vi "PJ1_สไลด์.vi"() -> ()   [LabVIEW 2024]
uses:
  <vilib>/express/express analysis/Spectral/XNode/ExpressSpectralMeasurementsBlockNode.xnode
  <vilib>/express/express analysis/Spectral/Block/exnSpectralBlock spectral measurements PSD poly.vi
  <vilib>/express/express analysis/Spectral/Block/exnSpectralBlock spectral measurements PSD DDT.vi
  <vilib>/Instr/_visa.llb/VISA Configure Serial Port (Instr).vi
panel:
  out "Numeric":i32
  in  "Upper Cut-Off":dbl=40.0
  out "PSD":dynamicdata(graph)
  out "PSD MAX":dbl
  out "Index ที่มากที่สุด":i32
  out "max value":dbl
  out "B 18+1":dbl
  out "N 18+1":dbl
  in  "Aj 18+1":dbl
  out "B 18+1":dbl
  out "PSD 18+1":dbl
  out "B 18":dbl
  out "N 18":dbl
  in  "Aj 18":dbl
  out "B 18":dbl
  out "PSD 18":dbl
  out "B 18-1":dbl
  out "N 18-1":dbl
  in  "Aj 18-1":dbl
  out "B 18-1":dbl
  out "PSD 18-1":dbl
  out "9 Hz":dbl[](array[numeric])
  out "Max Index 9":i32
  out "PSD max 9":dbl
  out "PSD 9-1":dbl
  out "B 9-1":dbl
  in  "Aj 9-1":dbl
  out "N 9-1":dbl
  out "B 9-1":dbl
  out "PSD 9":dbl
  out "B 9":dbl
  in  "Aj 9":dbl
  out "N 9":dbl
  out "B 9":dbl
  out "PSD 9+1":dbl
  out "B 9+1":dbl
  in  "Aj 9+1":dbl
  out "N 9+1":dbl
  out "B 9+1":dbl
  out "8 Hz":dbl[](array[numeric])
  out "Max Index 8":i32
  out "PSD max 8":dbl
  out "B 16+1":dbl
  out "N 16+1":dbl
  in  "Aj  16+1":dbl
  out "B 16+1":dbl
  out "PSD  16+1":dbl
  out "B 16":dbl
  out "N  16":dbl
  in  "Aj  16":dbl
  out "B 16":dbl
  out "PSD  16":dbl
  out "B 16-1":dbl
  out "N  16-1":dbl
  in  "Aj   16-1":dbl
  out "B   16-1":dbl
  out "PSD 16-1":dbl
  out "B 8+1":dbl
  out "N 8+1":dbl
  in  "Aj  8+1":dbl
  out "B  8+1":dbl
  out "PSD 8+1":dbl
  out "B 8":dbl
  out "N  8":dbl
  in  "Aj  8":dbl
  out "B  8":dbl
  out "PSD 8":dbl
  out "B 8-1":dbl
  out "N  8-1":dbl
  in  "Aj  8-1":dbl
  out "B  8-1":dbl
  out "PSD 8-1":dbl
  out "PSD 14+1":dbl
  out "B 14+1":dbl
  in  "Aj 14+1":dbl
  out "N 14+1":dbl
  out "B 14+1":dbl
  out "PSD 14":dbl
  out "B 14":dbl
  in  "Aj 14":dbl
  out "N 14":dbl
  out "B 14":dbl
  out "PSD 14-1":dbl
  out "B 14-1":dbl
  in  "Aj 14-1":dbl
  out "N 14-1":dbl
  out "B 14-1":dbl
  out "PSD7+1":dbl
  out "B7+1":dbl
  in  "Aj7+1":dbl
  out "N7+1":dbl
  out "B7+1":dbl
  out "PSD 7":dbl
  out "B 7":dbl
  in  "Aj 7":dbl
  out "N7":dbl
  out "B7":dbl
  out "7 Hz":dbl[](array[numeric])
  out "Max Index 7":i32
  out "PSD max 7":dbl
  out "PSD 7-1":dbl
  out "B 7-1":dbl
  in  "Aj 7-1":dbl
  out "N7-1":dbl
  out "B7-1":dbl
  out "B12-1":dbl
  out "N12-1":dbl
  in  "Aj 12-1":dbl
  out "B 12-1":dbl
  out "PSD 12-1":dbl
  out "B12":dbl
  out "N12":dbl
  in  "Aj 12":dbl
  out "B12":dbl
  out "PSD 12":dbl
  out "B12+1":dbl
  out "N12+1":dbl
  in  "Aj 12+1":dbl
  out "B 12+1":dbl
  out "PSD 12+1":dbl
  out "B6+1":dbl
  out "N6+1":dbl
  in  "Aj 6+1":dbl
  out "B 6+1":dbl
  out "PSD 6+1":dbl
  out "B6":dbl
  out "N6":dbl
  in  "Aj 6":dbl
  out "B6":dbl
  out "PSD 6":dbl
  out "PSD 6-1":dbl
  out "6 Hz":dbl[](array[numeric])
  out "Max Index 6":i32
  out "PSD max 6":dbl
  out "B 6-1":dbl
  in  "Aj 6-1":dbl
  out "N6-1":dbl
  out "B6-1":dbl
  in  "Baseline":bool
  out "appended array":dbl[][](array[numeric])
  out "Filtered Signal":dynamicdata(graph)
  in  "Lower Cut-Off":dbl=1.0
  out "data":dynamicdata(graph) caption="Raw Data"
  in  "number of samples":i32=1000
  in  "rate":dbl=200.0 min=200.0 max=200.0
  out "?":bool
  out "?":bool
  out "?":bool
  out "?":bool
  out "?":bool
  out "?":bool
  out "?":bool
  out "?":bool
  out "?":bool
  out "?":bool
  out "?":bool=TRUE
  out "?":bool=TRUE
  out "?":bool=TRUE
  out "?":bool=TRUE
  out "?":bool=TRUE
  out "?":bool=TRUE
  out "?":bool=TRUE
  out "?":bool=TRUE
  out "?":bool=TRUE
  out "?":bool=TRUE
  out "?":bool
  out "?":bool
  out "?":bool
  out "?":bool
  out "?":bool
  out "?":bool
  out "?":bool
  out "?":bool
  out "?":bool
  out "?":bool
  out "?":bool=TRUE
  out "?":bool=TRUE
  out "?":bool=TRUE
  out "?":bool=TRUE
  out "?":bool=TRUE
  out "?":bool=TRUE
  out "?":bool=TRUE
  out "?":bool=TRUE
  out "?":bool=TRUE
  out "?":bool=TRUE
  out "?":bool
  out "?":bool
  out "?":bool
  out "?":bool
  out "?":bool
  out "?":bool
  out "?":bool
  out "?":bool
  out "?":bool
  out "?":bool
  out "?":bool=TRUE
  out "?":bool=TRUE
  out "?":bool=TRUE
  out "?":bool=TRUE
  out "?":bool=TRUE
  out "?":bool=TRUE
  out "?":bool=TRUE
  out "?":bool=TRUE
  out "?":bool=TRUE
  out "?":bool=TRUE
  out "?":bool
  out "?":bool
  out "?":bool
  out "?":bool
  out "?":bool
  out "?":bool
  out "?":bool
  out "?":bool
  out "?":bool
  out "?":bool
  out "?":bool=TRUE
  out "?":bool=TRUE
  out "?":bool=TRUE
  out "?":bool=TRUE
  out "?":bool=TRUE
  out "?":bool=TRUE
  out "?":bool=TRUE
  out "?":bool=TRUE
  out "?":bool=TRUE
  out "?":bool=TRUE
  out "9 HZ":bool
  out "8 HZ":bool
  out "6 HZ":bool
  out "7 HZ":bool
  in  "Tab Control":enum32{"MENU", "COMMU", "CALL", "ELEC"}(tab)
  out "555":bool
  in  "ELEC":bool
  in  "MENU 3":bool
  in  "CALL":bool
  in  "COMMU":bool
  in  "start":bool
  in  "Text3":bool
  in  "Text2":bool
  out "String":string
  in  "Text1":bool
  in  "send":bool
  in  "Back 2":bool
  in  "Back 3":bool
  in  "1 3":bool
  in  "1 2":bool
  in  "1":bool
  out "String 2":string
  in  "SOS CALLING":bool
  in  "Blank Button 14":bool
  in  "LED":bool
  in  "Blank Button 12":bool
  in  "Back 4":bool
  in  "VISA resource name":refnum<visa-resource-name>
  # "Tel."
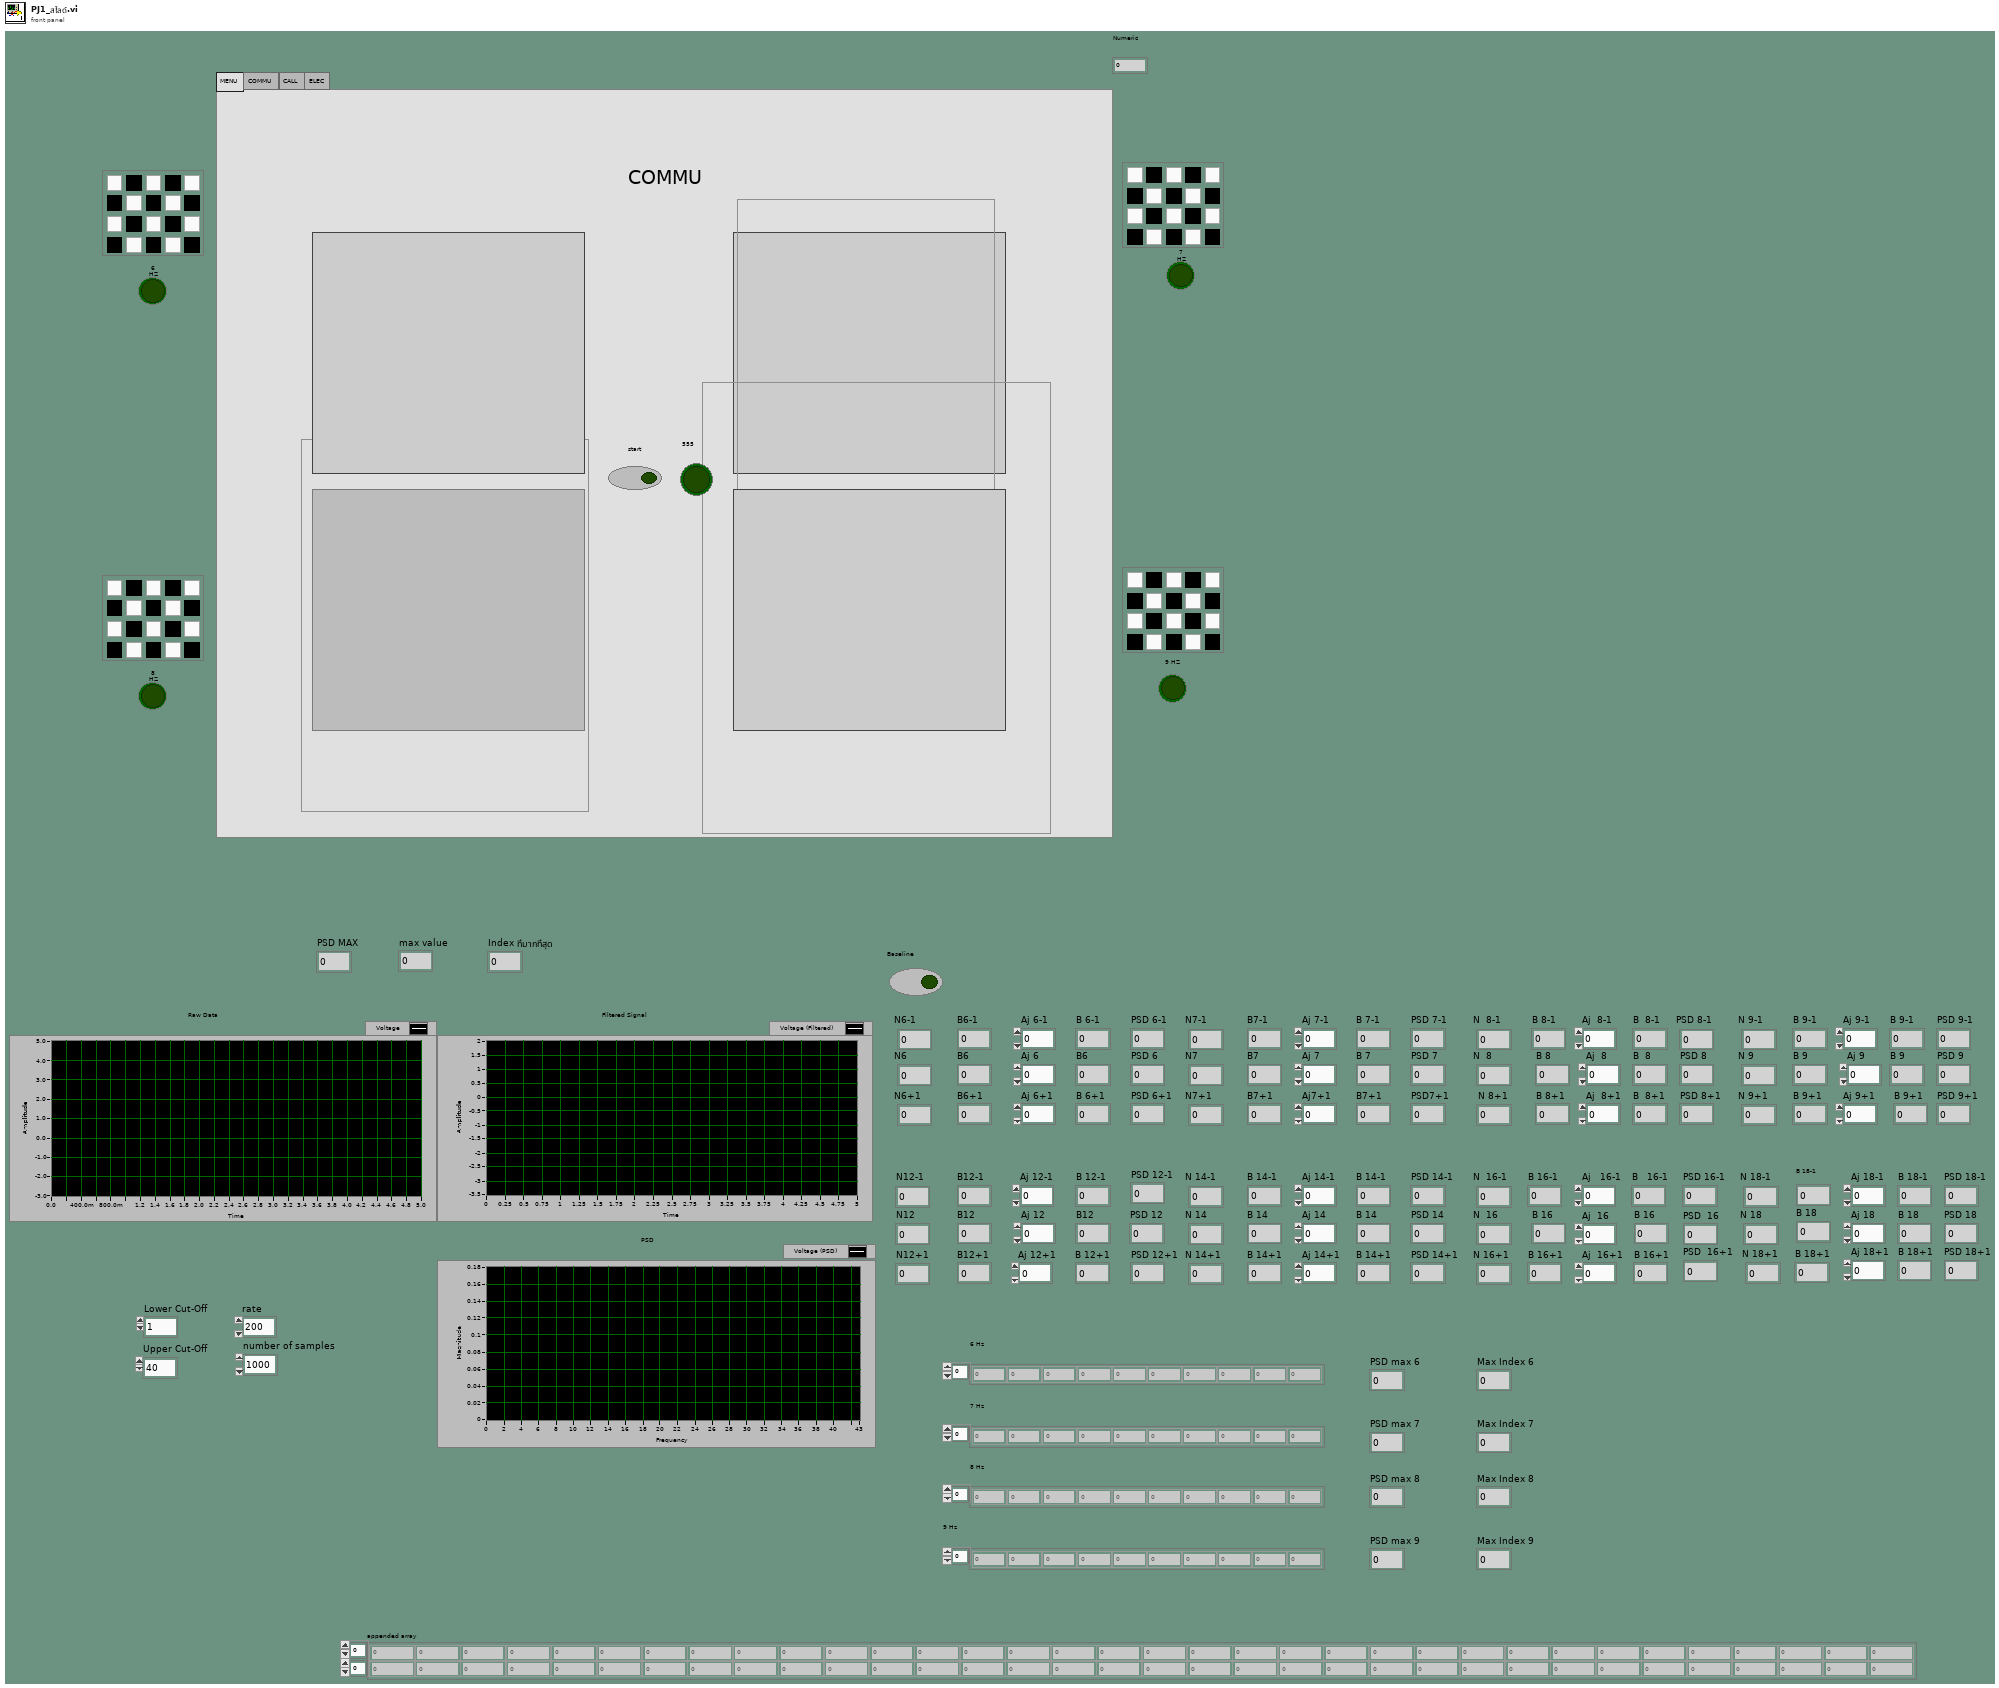
[diagram p1: front panel]
types:
  T1 = cluster{"averaging mode":u16, "weighting mode":u16, "number of averages":u32}
  T2 = cluster{"dB On (F)":bool, "unwrap phase (F)":bool, "convert to degree (F)":bool}
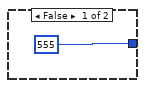
[diagram p3: hidden frame]
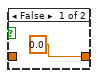
[diagram p4: hidden frame]
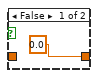
[diagram p6: hidden frame]
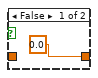
[diagram p8: hidden frame]
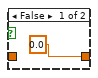
[diagram p10: hidden frame]
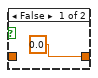
[diagram p12: hidden frame]
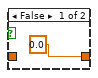
[diagram p14: hidden frame]
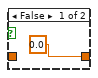
[diagram p16: hidden frame]
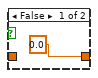
[diagram p18: hidden frame]
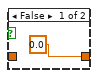
[diagram p20: hidden frame]
diagram:
  (unwired) FALSE
  n1 = while {
    stop <- FALSE stop-if-true
    n2 = event shown="[1] \"COMMU\": Value Change" {
      selector: _ -> [_ _ _ _ _ _ _]
      dyn-events: _ -> [_ _ _ _ _ _ _]
      timeout: _ -> [_ _ _ _ _ _ _]
      event Timeout {
        n3 = event-data() -> ()  [unwired: 1 in, 3 out]
      }
      event "COMMU": Value Change {
        n4 = event-data() -> ()  [unwired: 1 in, 6 out]
        n5 = local write "Tab Control"(enum32{"TAB 1", "TAB 2", "TAB 3", "TAB 4"}."TAB 2" ("Tab Control")) -> ()
      }
      event #2 (no event record) {
        n6 = event-data() -> ()  [unwired: 1 in, 6 out]
        n7 = local write "Tab Control"(enum32{"TAB 1", "TAB 2", "TAB 3", "TAB 4"}."TAB 1" ("Tab Control")) -> ()
      }
      event "CALL": Value Change {
        n8 = event-data() -> ()  [unwired: 1 in, 6 out]
        n9 = local write "Tab Control"(enum32{"TAB 1", "TAB 2", "TAB 3", "TAB 4"}."TAB 3" ("Tab Control")) -> ()
      }
      event "MENU 3": Value Change {
        n10 = event-data() -> ()  [unwired: 1 in, 6 out]
        n11 = local write "Tab Control"(enum32{"TAB 1", "TAB 2", "TAB 3", "TAB 4"}."TAB 4" ("Tab Control")) -> ()
      }
      event "ELEC": Value Change {
        n12 = event-data() -> ()  [unwired: 1 in, 6 out]
        n13 = local write "Tab Control"(enum32{"TAB 1", "TAB 2", "TAB 3", "TAB 4"}."TAB 4" ("Tab Control")) -> ()
      }
      event "Back 4": Value Change {
        n14 = event-data() -> ()  [unwired: 1 in, 6 out]
        n15 = local write "Tab Control"(enum32{"TAB 1", "TAB 2", "TAB 3", "TAB 4"}."TAB 1" ("Tab Control")) -> ()
      }
    }
  }
  n16 = while {
    shift-right: [w16] -> _
    shift-left: "" -> [w18]
    stop <- FALSE stop-if-true
    n17 = event shown="[3] \"Back 3\": Value Change" {
      selector: _ -> [_ _ _ _]
      dyn-events: _ -> [_ _ _ _]
      timeout: _ -> [_ _ _ _]
      tunnel: w18 -> [_ _ _ _]
      tunnel: ["0622436287" "1669" " 0937529340" _] -> w16
      event "1 2": Value Change {
        n18 = event-data() -> ()  [unwired: 1 in, 6 out]
      }
      event "1": Value Change {
        n19 = event-data() -> ()  [unwired: 1 in, 6 out]
      }
      event "1 3": Value Change {
        n20 = event-data() -> ()  [unwired: 1 in, 6 out]
      }
      event "Back 3": Value Change {
        n21 = event-data() -> ()  [unwired: 1 in, 6 out]
        n22 = local write "Tab Control"(enum32{"TAB 1", "TAB 2", "TAB 3", "TAB 4"}."TAB 1" ("Tab Control")) -> ()
      }
    }
    "String 2" <- w16
  }
  n23 = case shown="True" {
    selector: _ -> [_ _]
    frame False {
    }
    frame True {
      n24 = while {
        stop <- FALSE stop-if-true
        n25 = call "DAQ Assistant2"("rate"="rate", "number of samples"="number of samples") -> ("data"=w405:dynamicdata)  [unwired: 15 in, 2 out]
        "data" <- w405
        n26 = Divide(x="rate", y="number of samples") -> (x/y=w112:dbl)
        n27 = call "Filter"("Lower Cut-Off"="Lower Cut-Off", "Upper Cut-Off"="Upper Cut-Off", "Signal"=w405) -> ("Filtered Signal"=w403:dynamicdata)  [unwired: 7 in, 1 out]
        "Filtered Signal" <- w403
        n28 = Divide(x=8.0, y=w112) -> (x/y=w212:dbl)
        n29 = Divide(x=16.0, y=w112) -> (x/y=w164:dbl)
        n30 = Divide(x=14.0, y=w112) -> (x/y=w237:dbl)
        n31 = Divide(x=18.0, y=w112) -> (x/y=w87:dbl)
        n32 = xnode "Spectral Measurements"("Signals"=w403) -> ("PSD"=w49:dynamicdata)  [unwired: 1 in, 1 out]
        "PSD" <- w49
        n33 = Divide(x=9.0, y=w112) -> (x/y=w130:dbl)
        n34 = Divide(x=7.0, y=w112) -> (x/y=w254:dbl)
        n35 = Divide(x=12.0, y=w112) -> (x/y=w323:dbl)
        n36 = Divide(x=6.0, y=w112) -> (x/y=w372:dbl)
        n37 = call "Convert from Dynamic Data"("Dynamic Data Type"=w49) -> ("Array"=w402:dbl[])  [unwired: 3 in]
        n38 = Decrement(x=w130) -> (x-1=w161:dbl)
        n39 = Increment(x=w130) -> (x+1=w129:dbl)
        n40 = Increment(x=w87) -> (x+1=w76:dbl)
        n41 = Decrement(x=w87) -> (x-1=w101:dbl)
        n42 = Decrement(x=w237) -> (x-1=w266:dbl)
        n43 = Increment(x=w212) -> (x+1=w202:dbl)
        n44 = Decrement(x=w164) -> (x-1=w187:dbl)
        n45 = Decrement(x=w372) -> (x-1=w385:dbl)
        n46 = Decrement(x=w254) -> (x-1=w295:dbl)
        "PSD 7-1" <- w295
        n47 = Increment(x=w254) -> (x+1=w280:dbl)
        n48 = Decrement(x=w212) -> (x-1=w225:dbl)
        n49 = Increment(x=w164) -> (x+1=w163:dbl)
        n50 = Increment(x=w372) -> (x+1=w361:dbl)
        n51 = Increment(x=w237) -> (x+1=w243:dbl)
        n52 = Decrement(x=w323) -> (x-1=w328:dbl)
        n53 = Increment(x=w323) -> (x+1=w322:dbl)
        n54 = Build Array(w402) -> (w77:dbl[][])
        "appended array" <- w77
        n55 = Index Array(array=w77, index (row)=0, index (col)=w187) -> (element=w198:dbl)
        "PSD 16-1" <- w198
        n56 = Index Array(array=w77, index (row)=0 ("disabled index (row)"), index (col)=w163) -> (element=w175:dbl)
        "PSD  16+1" <- w175
        n57 = Index Array(array=w77, index (row)=0 ("disabled index (row)"), index (col)=w164) -> (element=w177:dbl)
        "PSD  16" <- w177
        n58 = Index Array(array=w77, index (row)=0, index (col)=w243) -> (element=w244:dbl)
        "PSD 14+1" <- w244
        n59 = Index Array(array=w77, index (row)=0 ("disabled index (row)"), index (col)=w101) -> (element=w99:dbl)
        "PSD 18-1" <- w99
        n60 = Index Array(array=w77, index (row)=0, index (col)=w202) -> (element=w200:dbl)
        "PSD 8+1" <- w200
        n61 = Index Array(array=w77, index (row)=0 ("disabled index (row)"), index (col)=w76) -> (element=w73:dbl)
        "PSD 18+1" <- w73
        n62 = Index Array(array=w77, index (row)=0, index (col)=w129) -> (element=w118:dbl)
        "PSD 9-1" <- w118
        n63 = Index Array(array=w77, index (row)=0, index (col)=w212) -> (element=w223:dbl)
        "PSD 8" <- w223
        n64 = Index Array(array=w77, index (row)=0 ("disabled index (row)"), index (col)=w87) -> (element=w88:dbl)
        "PSD 18" <- w88
        n65 = Index Array(array=w77, index (row)=0, index (col)=w225) -> (element=w224:dbl)
        "PSD 8-1" <- w224
        n66 = Index Array(array=w77, index (row)=0, index (col)=w130) -> (element=w131:dbl)
        "PSD 9" <- w131
        n67 = Index Array(array=w77, index (row)=0, index (col)=w161) -> (element=w142:dbl)
        "PSD 9+1" <- w142
        n68 = Index Array(array=w77, index (row)=0, index (col)=w266) -> (element=w268:dbl)
        "PSD 14-1" <- w268
        n69 = Index Array(array=w77, index (row)=0, index (col)=w237) -> (element=w255:dbl)
        "PSD 14" <- w255
        n70 = Index Array(array=w77, index (row)=0, index (col)=w295) -> ()  [unwired: 1 out]
        n71 = Index Array(array=w77, index (row)=0 ("disabled index (row)"), index (col)=w254) -> (element=w292:dbl)
        "PSD 7" <- w292
        n72 = Index Array(array=w77, index (row)=0, index (col)=w280) -> (element=w281:dbl)
        "PSD7+1" <- w281
        n73 = Index Array(array=w77, index (row)=0 ("disabled index (row)"), index (col)=w361) -> (element=w359:dbl)
        "PSD 6+1" <- w359
        n74 = Index Array(array=w77, index (row)=0, index (col)=w328) -> (element=w327:dbl)
        "PSD 12-1" <- w327
        n75 = Index Array(array=w77, index (row)=0 ("disabled index (row)"), index (col)=w323) -> (element=w324:dbl)
        "PSD 12" <- w324
        n76 = Index Array(array=w77, index (row)=0 ("disabled index (row)"), index (col)=w322) -> (element=w320:dbl)
        "PSD 12+1" <- w320
        n77 = Index Array(array=w77, index (row)=0, index (col)=w372) -> (element=w373:dbl)
        "PSD 6" <- w373
        n78 = Index Array(array=w77, index (row)=0, index (col)=w385) -> (element=w392:dbl)
        "PSD 6-1" <- w392
        n79 = feedback #1() -> (w25:dbl)  [unwired: 1 in]
        "B 18" <- w25
        n80 = case shown="False" "Baseline" {
          tunnel: w88 -> [_ w415]
          tunnel: [w414 w415] -> w90
          tunnel: w25 -> [w414 _]
          frame False {
          }
          frame True {
          }
        }
        n81 = feedback-in #1(w90) -> ()
        n82 = feedback #2() -> (w26:dbl)  [unwired: 1 in]
        "B 18-1" <- w26
        n83 = case shown="False" "Baseline" {
          tunnel: w99 -> [_ w419]
          tunnel: [w418 w419] -> w110
          tunnel: w26 -> [w418 _]
          frame False {
          }
          frame True {
          }
        }
        n84 = feedback-in #2(w110) -> ()
        n85 = feedback #3() -> (w24:dbl)  [unwired: 1 in]
        "B 18+1" <- w24
        n86 = case shown="False" "Baseline" {
          tunnel: w73 -> [_ w411]
          tunnel: [w410 w411] -> w86
          tunnel: w24 -> [w410 _]
          frame False {
          }
          frame True {
          }
        }
        n87 = feedback-in #3(w86) -> ()
        n88 = feedback #4() -> (w32:dbl)  [unwired: 1 in]
        "B 16-1" <- w32
        n89 = case shown="True" "Baseline" {
          tunnel: w198 -> [_ w443]
          tunnel: [w442 w443] -> w188
          tunnel: w32 -> [w442 _]
          frame False {
          }
          frame True {
          }
        }
        n90 = feedback-in #4(w188) -> ()
        n91 = feedback #5() -> (w30:dbl)  [unwired: 1 in]
        "B 16+1" <- w30
        n92 = case shown="True" "Baseline" {
          tunnel: w175 -> [_ w435]
          tunnel: [w434 w435] -> w166
          tunnel: w30 -> [w434 _]
          frame False {
          }
          frame True {
          }
        }
        n93 = feedback-in #5(w166) -> ()
        n94 = feedback #6() -> (w31:dbl)  [unwired: 1 in]
        "B 16" <- w31
        n95 = case shown="True" "Baseline" {
          tunnel: w177 -> [_ w439]
          tunnel: [w438 w439] -> w186
          tunnel: w31 -> [w438 _]
          frame False {
          }
          frame True {
          }
        }
        n96 = feedback-in #6(w186) -> ()
        n97 = feedback #7() -> (w33:dbl)  [unwired: 1 in]
        "B 8+1" <- w33
        n98 = case shown="True" "Baseline" {
          tunnel: w200 -> [_ w447]
          tunnel: [w446 w447] -> w211
          tunnel: w33 -> [w446 _]
          frame False {
          }
          frame True {
          }
        }
        n99 = feedback-in #7(w211) -> ()
        n100 = feedback #8() -> (w36:dbl)  [unwired: 1 in]
        "B 14+1" <- w36
        n101 = case shown="True" "Baseline" {
          tunnel: w244 -> [_ w459]
          tunnel: [w458 w459] -> w245
          tunnel: w36 -> [w458 _]
          frame False {
          }
          frame True {
          }
        }
        n102 = feedback-in #8(w245) -> ()
        n103 = feedback #9() -> (w34:dbl)  [unwired: 1 in]
        "B 8" <- w34
        n104 = case shown="True" "Baseline" {
          tunnel: w223 -> [_ w451]
          tunnel: [w450 w451] -> w214
          tunnel: w34 -> [w450 _]
          frame False {
          }
          frame True {
          }
        }
        n105 = feedback-in #9(w214) -> ()
        n106 = feedback #10() -> (w28:dbl)  [unwired: 1 in]
        "B 9" <- w28
        n107 = case shown="False" "Baseline" {
          tunnel: w131 -> [_ w427]
          tunnel: [w426 w427] -> w132
          tunnel: w28 -> [w426 _]
          frame False {
          }
          frame True {
          }
        }
        n108 = feedback-in #10(w132) -> ()
        n109 = feedback #11() -> (w35:dbl)  [unwired: 1 in]
        "B 8-1" <- w35
        n110 = case shown="True" "Baseline" {
          tunnel: w224 -> [_ w455]
          tunnel: [w454 w455] -> w235
          tunnel: w35 -> [w454 _]
          frame False {
          }
          frame True {
          }
        }
        n111 = feedback-in #11(w235) -> ()
        n112 = feedback #12() -> (w29:dbl)  [unwired: 1 in]
        "B 9+1" <- w29
        n113 = case shown="True" "Baseline" {
          tunnel: w142 -> [_ w431]
          tunnel: [w430 w431] -> w143
          tunnel: w29 -> [w430 _]
          frame False {
          }
          frame True {
          }
        }
        n114 = feedback-in #12(w143) -> ()
        n115 = feedback #13() -> (w44:dbl)  [unwired: 1 in]
        "B12-1" <- w44
        n116 = case shown="True" "Baseline" {
          tunnel: w327 -> [_ w491]
          tunnel: [w490 w491] -> w339
          tunnel: w44 -> [w490 _]
          frame False {
          }
          frame True {
          }
        }
        n117 = feedback-in #13(w339) -> ()
        n118 = feedback #14() -> (w38:dbl)  [unwired: 1 in]
        "B 14-1" <- w38
        n119 = case shown="True" "Baseline" {
          tunnel: w268 -> [_ w467]
          tunnel: [w466 w467] -> w269
          tunnel: w38 -> [w466 _]
          frame False {
          }
          frame True {
          }
        }
        n120 = feedback-in #14(w269) -> ()
        n121 = feedback #15() -> (w27:dbl)  [unwired: 1 in]
        "B 9-1" <- w27
        n122 = case shown="False" "Baseline" {
          tunnel: w118 -> [_ w423]
          tunnel: [w422 w423] -> w119
          tunnel: w27 -> [w422 _]
          frame False {
          }
          frame True {
          }
        }
        n123 = feedback-in #15(w119) -> ()
        n124 = feedback #16() -> (w45:dbl)  [unwired: 1 in]
        "B6+1" <- w45
        n125 = case shown="True" "Baseline" {
          tunnel: w359 -> [_ w495]
          tunnel: [w494 w495] -> w362
          tunnel: w45 -> [w494 _]
          frame False {
          }
          frame True {
          }
        }
        n126 = feedback-in #16(w362) -> ()
        n127 = feedback #17() -> (w46:dbl)  [unwired: 1 in]
        "B6" <- w46
        n128 = case shown="True" "Baseline" {
          tunnel: w373 -> [_ w499]
          tunnel: [w498 w499] -> w383
          tunnel: w46 -> [w498 _]
          frame False {
          }
          frame True {
          }
        }
        n129 = feedback-in #17(w383) -> ()
        n130 = feedback #18() -> (w47:dbl)  [unwired: 1 in]
        "B6-1" <- w47
        n131 = case shown="True" "Baseline" {
          tunnel: w392 -> [_ w503]
          tunnel: [w502 w503] -> w384
          tunnel: w47 -> [w502 _]
          frame False {
          }
          frame True {
          }
        }
        n132 = feedback-in #18(w384) -> ()
        n133 = feedback #19() -> (w37:dbl)  [unwired: 1 in]
        "B 14" <- w37
        n134 = case shown="True" "Baseline" {
          tunnel: w255 -> [_ w463]
          tunnel: [w462 w463] -> w257
          tunnel: w37 -> [w462 _]
          frame False {
          }
          frame True {
          }
        }
        n135 = feedback-in #19(w257) -> ()
        n136 = feedback #20() -> (w42:dbl)  [unwired: 1 in]
        "B12+1" <- w42
        n137 = case shown="True" "Baseline" {
          tunnel: w320 -> [_ w483]
          tunnel: [w482 w483] -> w357
          tunnel: w42 -> [w482 _]
          frame False {
          }
          frame True {
          }
        }
        n138 = feedback-in #20(w357) -> ()
        n139 = Add(x=w25, y="Aj 18") -> (x+y=w94:dbl)
        "B 18" <- w94
        n140 = Add(x=w26, y="Aj 18-1") -> (x+y=w106:dbl)
        "B 18-1" <- w106
        n141 = Add(x=w24, y="Aj 18+1") -> (x+y=w82:dbl)
        "B 18+1" <- w82
        n142 = feedback #21() -> (w43:dbl)  [unwired: 1 in]
        "B12" <- w43
        n143 = case shown="True" "Baseline" {
          tunnel: w324 -> [_ w487]
          tunnel: [w486 w487] -> w340
          tunnel: w43 -> [w486 _]
          frame False {
          }
          frame True {
          }
        }
        n144 = feedback-in #21(w340) -> ()
        n145 = Add(x=w32, y="Aj   16-1") -> (x+y=w192:dbl)
        "B   16-1" <- w192
        n146 = Add(x=w30, y="Aj  16+1") -> (x+y=w170:dbl)
        "B 16+1" <- w170
        n147 = Add(x=w31, y="Aj  16") -> (x+y=w182:dbl)
        "B 16" <- w182
        n148 = Add(x=w33, y="Aj  8+1") -> (x+y=w207:dbl)
        "B  8+1" <- w207
        n149 = Add(x=w36, y="Aj 14+1") -> (x+y=w249:dbl)
        "B 14+1" <- w249
        n150 = Add(x=w34, y="Aj  8") -> (x+y=w218:dbl)
        "B  8" <- w218
        n151 = Add(x=w28, y="Aj 9") -> (x+y=w136:dbl)
        "B 9" <- w136
        n152 = Add(x=w35, y="Aj  8-1") -> (x+y=w231:dbl)
        "B  8-1" <- w231
        n153 = Add(x=w29, y="Aj 9+1") -> (x+y=w147:dbl)
        "B 9+1" <- w147
        n154 = Add(x=w44, y="Aj 12-1") -> (x+y=w335:dbl)
        "B 12-1" <- w335
        n155 = Add(x=w38, y="Aj 14-1") -> (x+y=w273:dbl)
        "B 14-1" <- w273
        n156 = Add(x=w27, y="Aj 9-1") -> (x+y=w123:dbl)
        "B 9-1" <- w123
        n157 = Multiply(x=w25, y=5.0) -> (x*y=w97:dbl)
        "N 18" <- w97
        n158 = Add(x=w45, y="Aj 6+1") -> (x+y=w366:dbl)
        "B 6+1" <- w366
        n159 = Multiply(x=w26, y=5.0) -> (x*y=w103:dbl)
        "N 18-1" <- w103
        n160 = Multiply(x=w24, y=5.0) -> (x*y=w79:dbl)
        "N 18+1" <- w79
        n161 = feedback #22() -> (w39:dbl)  [unwired: 1 in]
        "B7+1" <- w39
        n162 = case shown="True" "Baseline" {
          tunnel: w281 -> [_ w471]
          tunnel: [w470 w471] -> w283
          tunnel: w39 -> [w470 _]
          frame False {
          }
          frame True {
          }
        }
        n163 = feedback-in #22(w283) -> ()
        n164 = feedback #23() -> (w40:dbl)  [unwired: 1 in]
        "B7" <- w40
        n165 = case shown="True" "Baseline" {
          tunnel: w292 -> [_ w475]
          tunnel: [w474 w475] -> w296
          tunnel: w40 -> [w474 _]
          frame False {
          }
          frame True {
          }
        }
        n166 = feedback-in #23(w296) -> ()
        n167 = Multiply(x=w32, y=5.0) -> (x*y=w195:dbl)
        "N  16-1" <- w195
        n168 = Multiply(x=w30, y=5.0) -> (x*y=w173:dbl)
        "N 16+1" <- w173
        n169 = Multiply(x=w31, y=5.0) -> (x*y=w179:dbl)
        "N  16" <- w179
        n170 = Multiply(x=w33, y=5.0) -> (x*y=w204:dbl)
        "N 8+1" <- w204
        n171 = feedback #24() -> (w41:dbl)  [unwired: 1 in]
        "B7-1" <- w41
        n172 = case shown="False" "Baseline" {
          tunnel: w295 -> [_ w479]
          tunnel: [w478 w479] -> w309
          tunnel: w41 -> [w478 _]
          frame False {
          }
          frame True {
          }
        }
        n173 = feedback-in #24(w309) -> ()
        n174 = Add(x=w46, y="Aj 6") -> (x+y=w379:dbl)
        "B6" <- w379
        n175 = Add(x=w47, y="Aj 6-1") -> (x+y=w393:dbl)
        "B 6-1" <- w393
        n176 = Add(x=w37, y="Aj 14") -> (x+y=w261:dbl)
        "B 14" <- w261
        n177 = Multiply(x=w36, y=5.0) -> (x*y=w252:dbl)
        "N 14+1" <- w252
        n178 = Multiply(x=w34, y=5.0) -> (x*y=w221:dbl)
        "N  8" <- w221
        n179 = Multiply(x=w28, y=5.0) -> (x*y=w139:dbl)
        "N 9" <- w139
        n180 = Multiply(x=w35, y=5.0) -> (x*y=w228:dbl)
        "N  8-1" <- w228
        n181 = Multiply(x=w29, y=5.0) -> (x*y=w150:dbl)
        "N 9+1" <- w150
        n182 = Add(x=w42, y="Aj 12+1") -> (x+y=w353:dbl)
        "B 12+1" <- w353
        n183 = Multiply(x=w44, y=5.0) -> (x*y=w332:dbl)
        "N12-1" <- w332
        n184 = Multiply(x=w38, y=5.0) -> (x*y=w276:dbl)
        "N 14-1" <- w276
        n185 = Add(x=w43, y="Aj 12") -> (x+y=w344:dbl)
        "B12" <- w344
        n186 = Multiply(x=w27, y=5.0) -> (x*y=w126:dbl)
        "N 9-1" <- w126
        n187 = Multiply(x=w45, y=5.0) -> (x*y=w369:dbl)
        "N6+1" <- w369
        n188 = Greater?(x=w88, y=w94) -> (0:w95:bool)
        n189 = Greater?(x=w99, y=w106) -> (0:w105:bool)
        n190 = Greater?(x=w73, y=w82) -> (0:w81:bool)
        n191 = Less?(x=w88, y=w97) -> (x < y?=w96:bool)
        n192 = Less?(x=w99, y=w103) -> (x < y?=w104:bool)
        n193 = Multiply(x=w46, y=5.0) -> (x*y=w376:dbl)
        "N6" <- w376
        n194 = Multiply(x=w47, y=5.0) -> (x*y=w396:dbl)
        "N6-1" <- w396
        n195 = Multiply(x=w37, y=5.0) -> (x*y=w264:dbl)
        "N 14" <- w264
        n196 = Greater?(x=w198, y=w192) -> (0:w193:bool)
        n197 = Less?(x=w73, y=w79) -> (x < y?=w80:bool)
        n198 = Greater?(x=w175, y=w170) -> (0:w171:bool)
        n199 = Greater?(x=w177, y=w182) -> (0:w181:bool)
        n200 = Greater?(x=w200, y=w207) -> (0:w206:bool)
        n201 = Less?(x=w198, y=w195) -> (x < y?=w194:bool)
        n202 = Less?(x=w175, y=w173) -> (x < y?=w172:bool)
        n203 = Multiply(x=w42, y=5.0) -> (x*y=w350:dbl)
        "N12+1" <- w350
        n204 = Less?(x=w177, y=w179) -> (x < y?=w180:bool)
        n205 = Greater?(x=w244, y=w249) -> (0:w250:bool)
        n206 = Less?(x=w200, y=w204) -> (x < y?=w205:bool)
        n207 = Greater?(x=w223, y=w218) -> (0:w219:bool)
        n208 = Greater?(x=w131, y=w136) -> (0:w137:bool)
        n209 = Multiply(x=w43, y=5.0) -> (x*y=w347:dbl)
        "N12" <- w347
        n210 = Add(x=w39, y="Aj7+1") -> (x+y=w287:dbl)
        "B7+1" <- w287
        n211 = Less?(x=w244, y=w252) -> (x < y?=w251:bool)
        n212 = Greater?(x=w224, y=w231) -> (0:w230:bool)
        n213 = Less?(x=w223, y=w221) -> (x < y?=w220:bool)
        n214 = Less?(x=w131, y=w139) -> (x < y?=w138:bool)
        n215 = Greater?(x=w142, y=w147) -> (0:w148:bool)
        n216 = Add(x=w40, y="Aj 7") -> (x+y=w300:dbl)
        "B 7" <- w300
        n217 = Less?(x=w224, y=w228) -> (x < y?=w229:bool)
        n218 = Greater?(x=w327, y=w335) -> (0:w334:bool)
        n219 = Greater?(x=w268, y=w273) -> (0:w274:bool)
        n220 = Less?(x=w142, y=w150) -> (x < y?=w149:bool)
        n221 = Greater?(x=w118, y=w123) -> (0:w124:bool)
        n222 = Add(x=w41, y="Aj 7-1") -> (x+y=w313:dbl)
        "B 7-1" <- w313
        n223 = Greater?(x=w359, y=w366) -> (0:w367:bool)
        n224 = Less?(x=w327, y=w332) -> (x < y?=w333:bool)
        n225 = Less?(x=w268, y=w276) -> (x < y?=w275:bool)
        n226 = Less?(x=w118, y=w126) -> (x < y?=w125:bool)
        n227 = Less?(x=w359, y=w369) -> (x < y?=w368:bool)
        n228 = And(x=w96, y=w95) -> (x .and. y?=w93:bool)
        n229 = Subtract(x=w88, y=w94) -> (x-y=w92:dbl)
        n230 = And(x=w104, y=w105) -> (x .and. y?=w107:bool)
        n231 = Greater?(x=w373, y=w379) -> (0:w378:bool)
        n232 = Subtract(x=w99, y=w106) -> (x-y=w108:dbl)
        n233 = Greater?(x=w392, y=w393) -> (0:w394:bool)
        n234 = Greater?(x=w255, y=w261) -> (0:w262:bool)
        n235 = And(x=w80, y=w81) -> (x .and. y?=w83:bool)
        n236 = Subtract(x=w73, y=w82) -> (x-y=w84:dbl)
        n237 = Less?(x=w373, y=w376) -> (x < y?=w377:bool)
        n238 = Less?(x=w392, y=w396) -> (x < y?=w395:bool)
        n239 = Less?(x=w255, y=w264) -> (x < y?=w263:bool)
        n240 = And(x=w194, y=w193) -> (x .and. y?=w191:bool)
        n241 = Multiply(x=w39, y=5.0) -> (x*y=w290:dbl)
        "N7+1" <- w290
        n242 = Subtract(x=w198, y=w192) -> (x-y=w190:dbl)
        n243 = And(x=w172, y=w171) -> (x .and. y?=w169:bool)
        n244 = Subtract(x=w175, y=w170) -> (x-y=w168:dbl)
        n245 = Greater?(x=w320, y=w353) -> (0:w352:bool)
        n246 = Multiply(x=w40, y=5.0) -> (x*y=w303:dbl)
        "N7" <- w303
        n247 = And(x=w180, y=w181) -> (x .and. y?=w183:bool)
        n248 = And(x=w205, y=w206) -> (x .and. y?=w208:bool)
        n249 = Subtract(x=w177, y=w182) -> (x-y=w184:dbl)
        n250 = Subtract(x=w200, y=w207) -> (x-y=w209:dbl)
        n251 = Greater?(x=w324, y=w344) -> (0:w345:bool)
        n252 = Less?(x=w320, y=w350) -> (x < y?=w351:bool)
        n253 = And(x=w251, y=w250) -> (x .and. y?=w248:bool)
        n254 = Subtract(x=w244, y=w249) -> (x-y=w247:dbl)
        n255 = Multiply(x=w41, y=5.0) -> (x*y=w316:dbl)
        "N7-1" <- w316
        n256 = And(x=w220, y=w219) -> (x .and. y?=w217:bool)
        n257 = Subtract(x=w223, y=w218) -> (x-y=w216:dbl)
        n258 = And(x=w138, y=w137) -> (x .and. y?=w135:bool)
        n259 = Subtract(x=w131, y=w136) -> (x-y=w134:dbl)
        n260 = Less?(x=w324, y=w347) -> (x < y?=w346:bool)
        n261 = And(x=w229, y=w230) -> (x .and. y?=w232:bool)
        n262 = Subtract(x=w224, y=w231) -> (x-y=w233:dbl)
        n263 = And(x=w149, y=w148) -> (x .and. y?=w146:bool)
        n264 = Subtract(x=w142, y=w147) -> (x-y=w145:dbl)
        n265 = And(x=w333, y=w334) -> (x .and. y?=w336:bool)
        n266 = Subtract(x=w327, y=w335) -> (x-y=w337:dbl)
        n267 = And(x=w275, y=w274) -> (x .and. y?=w272:bool)
        n268 = Subtract(x=w268, y=w273) -> (x-y=w271:dbl)
        n269 = And(x=w125, y=w124) -> (x .and. y?=w122:bool)
        n270 = Subtract(x=w118, y=w123) -> (x-y=w121:dbl)
        n271 = Subtract(x=w359, y=w366) -> (x-y=w364:dbl)
        n272 = And(x=w368, y=w367) -> (x .and. y?=w365:bool)
        n273 = And(x=w395, y=w394) -> (x .and. y?=w391:bool)
        n274 = Subtract(x=w373, y=w379) -> (x-y=w381:dbl)
        n275 = And(x=w263, y=w262) -> (x .and. y?=w260:bool)
        n276 = Subtract(x=w392, y=w393) -> (x-y=w390:dbl)
        n277 = Greater?(x=w281, y=w287) -> (0:w288:bool)
        n278 = Subtract(x=w255, y=w261) -> (x-y=w259:dbl)
        n279 = Greater?(x=w292, y=w300) -> (0:w301:bool)
        n280 = And(x=w377, y=w378) -> (x .and. y?=w380:bool)
        n281 = Less?(x=w281, y=w290) -> (x < y?=w289:bool)
        n282 = Less?(x=w292, y=w303) -> (x < y?=w302:bool)
        n283 = Subtract(x=w320, y=w353) -> (x-y=w355:dbl)
        n284 = Greater?(x=w295, y=w313) -> (0:w314:bool)
        n285 = Subtract(x=w324, y=w344) -> (x-y=w342:dbl)
        n286 = And(x=w351, y=w352) -> (x .and. y?=w354:bool)
        n287 = Less?(x=w295, y=w316) -> (x < y?=w315:bool)
        n288 = And(x=w346, y=w345) -> (x .and. y?=w343:bool)
        n289 = And(x=w289, y=w288) -> (x .and. y?=w286:bool)
        n290 = Subtract(x=w281, y=w287) -> (x-y=w285:dbl)
        n291 = And(x=w302, y=w301) -> (x .and. y?=w299:bool)
        n292 = Subtract(x=w292, y=w300) -> (x-y=w298:dbl)
        n293 = And(x=w315, y=w314) -> (x .and. y?=w312:bool)
        n294 = Subtract(x=w295, y=w313) -> (x-y=w311:dbl)
        n295 = case shown="True" w336 {
          tunnel: w337 -> [_ w489]
          tunnel: [0.0 w489] -> w326
          frame False {
          }
          frame True {
          }
        }
        n296 = case shown="True" w365 {
          tunnel: w364 -> [_ w493]
          tunnel: [0.0 w493] -> w358
          frame False {
          }
          frame True {
          }
        }
        n297 = case shown="False" w391 {
          tunnel: w390 -> [_ w501]
          tunnel: [0.0 w501] -> w388
          frame False {
          }
          frame True {
          }
        }
        n298 = case shown="False" w380 {
          tunnel: w381 -> [_ w497]
          tunnel: [0.0 w497] -> w371
          frame False {
          }
          frame True {
          }
        }
        n299 = case shown="True" w354 {
          tunnel: w355 -> [_ w481]
          tunnel: [0.0 w481] -> w318
          frame False {
          }
          frame True {
          }
        }
        n300 = case shown="True" w93 {
          tunnel: w92 -> [_ w413]
          tunnel: [0.0 w413] -> w71
          frame False {
          }
          frame True {
          }
        }
        n301 = case shown="True" w343 {
          tunnel: w342 -> [_ w485]
          tunnel: [0.0 w485] -> w319
          frame False {
          }
          frame True {
          }
        }
        n302 = case shown="True" w107 {
          tunnel: w108 -> [_ w417]
          tunnel: [0.0 w417] -> w72
          frame False {
          }
          frame True {
          }
        }
        n303 = case shown="True" w83 {
          tunnel: w84 -> [_ w409]
          tunnel: [0.0 w409] -> w70
          frame False {
          }
          frame True {
          }
        }
        n304 = case shown="True" w191 {
          tunnel: w190 -> [_ w441]
          tunnel: [0.0 w441] -> w154
          frame False {
          }
          frame True {
          }
        }
        n305 = case shown="True" w169 {
          tunnel: w168 -> [_ w433]
          tunnel: [0.0 w433] -> w152
          frame False {
          }
          frame True {
          }
        }
        n306 = case shown="True" w183 {
          tunnel: w184 -> [_ w437]
          tunnel: [0.0 w437] -> w153
          frame False {
          }
          frame True {
          }
        }
        n307 = case shown="True" w208 {
          tunnel: w209 -> [_ w445]
          tunnel: [0.0 w445] -> w155
          frame False {
          }
          frame True {
          }
        }
        n308 = case shown="True" w248 {
          tunnel: w247 -> [_ w457]
          tunnel: [0.0 w457] -> w239
          frame False {
          }
          frame True {
          }
        }
        n309 = case shown="True" w217 {
          tunnel: w216 -> [_ w449]
          tunnel: [0.0 w449] -> w156
          frame False {
          }
          frame True {
          }
        }
        n310 = case shown="True" w260 {
          tunnel: w259 -> [_ w461]
          tunnel: [0.0 w461] -> w240
          frame False {
          }
          frame True {
          }
        }
        n311 = case shown="True" w135 {
          tunnel: w134 -> [_ w425]
          tunnel: [0.0 w425] -> w114
          frame False {
          }
          frame True {
          }
        }
        n312 = case shown="True" w232 {
          tunnel: w233 -> [_ w453]
          tunnel: [0.0 w453] -> w157
          frame False {
          }
          frame True {
          }
        }
        n313 = case shown="True" w272 {
          tunnel: w271 -> [_ w465]
          tunnel: [0.0 w465] -> w241
          frame False {
          }
          frame True {
          }
        }
        n314 = case shown="True" w286 {
          tunnel: w285 -> [_ w469]
          tunnel: [0.0 w469] -> w278
          frame False {
          }
          frame True {
          }
        }
        n315 = case shown="True" w146 {
          tunnel: w145 -> [_ w429]
          tunnel: [0.0 w429] -> w115
          frame False {
          }
          frame True {
          }
        }
        n316 = case shown="True" w299 {
          tunnel: w298 -> [_ w473]
          tunnel: [0.0 w473] -> w279
          frame False {
          }
          frame True {
          }
        }
        n317 = case shown="True" w122 {
          tunnel: w121 -> [_ w421]
          tunnel: [0.0 w421] -> w113
          frame False {
          }
          frame True {
          }
        }
        n318 = case shown="False" w312 {
          tunnel: w311 -> [_ w477]
          tunnel: [0.0 w477] -> w305
          frame False {
          }
          frame True {
          }
        }
        n319 = Build Array(w305, w279, w278, w241, w240, w239) -> (w306:dbl[])
        "7 Hz" <- w306
        n320 = Build Array(w388, w371, w358, w326, w319, w318) -> (w386:dbl[])
        "6 Hz" <- w386
        n321 = Array Max & Min(array=w306) -> (max value=w69:dbl, max index (indices)=→"Max Index 7":i32)  [unwired: 2 out]
        "PSD max 7" <- w69
        n322 = Array Max & Min(array=w386) -> (max value=w66:dbl, max index (indices)=→"Max Index 6":i32)  [unwired: 2 out]
        "PSD max 6" <- w66
        n323 = Build Array(w157, w156, w155, w154, w153, w152) -> (w158:dbl[])
        "8 Hz" <- w158
        n324 = Build Array(w115, w114, w113, w72, w71, w70) -> (w116:dbl[])
        "9 Hz" <- w116
        n325 = Array Max & Min(array=w158) -> (max value=w68:dbl, max index (indices)=→"Max Index 8":i32)  [unwired: 2 out]
        "PSD max 8" <- w68
        n326 = Array Max & Min(array=w116) -> (max value=w67:dbl, max index (indices)=→"Max Index 9":i32)  [unwired: 2 out]
        "PSD max 9" <- w67
        n327 = Build Array(w66, w69, w68, w67) -> (w65:dbl[])
        n328 = Array Max & Min(array=w65) -> (max value=w63:dbl, max index (indices)=w64:i32)  [unwired: 2 out]
        "max value" <- w63
        "PSD MAX" <- w63
        n329 = Greater?(x=w63, y=0.0 ("x")) -> (0:w61:bool)
        n330 = case shown="True" w61 {
          tunnel: w64 -> [_ w407]
          tunnel: [555 w407] -> w50
          frame False {
          }
          frame True {
          }
        }
        "Index ที่มากที่สุด" <- w50
        "Numeric" <- w50
        n331 = Equal?(x=0, y=w50) -> (x = y?=→"6 HZ":bool)
        n332 = Equal?(x=1, y=w50) -> (x = y?=→"7 HZ":bool)
        n333 = Equal?(x=2, y=w50) -> (x = y?=→"9 HZ":bool)
        n334 = Equal?(x=3, y=w50) -> (x = y?=→"8 HZ":bool)
        n335 = Equal?(x=555, y=w50) -> (x = y?=→"555":bool)
      }
    }
  }
  n336 = while {
    tunnel: ["start"] -> _
    stop <- FALSE stop-if-true
    n337 = while {
      stop <- FALSE stop-if-true
      w552 = 83.3333
      # "6 HZ"
      n338 = for {
        N: 2 -> [_]
        tunnel: w552 -> [w560]
        i -> [w561]
        n339 = Wait (ms)(milliseconds to wait=w560) -> ()  [unwired: 1 out]
        n340 = Equal?(x=1, y=w561) -> (x = y?=→"?" →"?" →"?" →"?" →"?" →"?" →"?" →"?" →"?" →"?":bool)
      }
      n341 = for {
        N: 2 -> [_]
        tunnel: w552 -> [w556]
        i -> [w558]
        n342 = Wait (ms)(milliseconds to wait=w556) -> ()  [unwired: 1 out]
        n343 = Equal?(x=0, y=w558) -> (x = y?=→"?" →"?" →"?" →"?" →"?" →"?" →"?" →"?" →"?" →"?":bool)
      }
    }
    n344 = while {
      stop <- FALSE stop-if-true
      w540 = 71.428571
      # "7 HZ"
      n345 = for {
        N: 2 -> [_]
        tunnel: w540 -> [w544]
        i -> [w546]
        n346 = Wait (ms)(milliseconds to wait=w544) -> ()  [unwired: 1 out]
        n347 = Equal?(x=0, y=w546) -> (x = y?=→"?" →"?" →"?" →"?" →"?" →"?" →"?" →"?" →"?" →"?":bool)
      }
      n348 = for {
        N: 2 -> [_]
        tunnel: w540 -> [w548]
        i -> [w549]
        n349 = Wait (ms)(milliseconds to wait=w548) -> ()  [unwired: 1 out]
        n350 = Equal?(x=1, y=w549) -> (x = y?=→"?" →"?" →"?" →"?" →"?" →"?" →"?" →"?" →"?" →"?":bool)
      }
    }
    n351 = while {
      stop <- FALSE stop-if-true
      w528 = 62.5
      # "8 HZ"
      n352 = for {
        N: 2 -> [_]
        tunnel: w528 -> [w536]
        i -> [w537]
        n353 = Wait (ms)(milliseconds to wait=w536) -> ()  [unwired: 1 out]
        n354 = Equal?(x=1, y=w537) -> (x = y?=→"?" →"?" →"?" →"?" →"?" →"?" →"?" →"?" →"?" →"?":bool)
      }
      n355 = for {
        N: 2 -> [_]
        tunnel: w528 -> [w532]
        i -> [w534]
        n356 = Wait (ms)(milliseconds to wait=w532) -> ()  [unwired: 1 out]
        n357 = Equal?(x=0, y=w534) -> (x = y?=→"?" →"?" →"?" →"?" →"?" →"?" →"?" →"?" →"?" →"?":bool)
      }
    }
    n358 = while {
      stop <- FALSE stop-if-true
      w516 = 55.5555
      # "9 HZ"
      n359 = for {
        N: 2 -> [_]
        tunnel: w516 -> [w524]
        i -> [w525]
        n360 = Wait (ms)(milliseconds to wait=w524) -> ()  [unwired: 1 out]
        n361 = Equal?(x=1, y=w525) -> (x = y?=→"?" →"?" →"?" →"?" →"?" →"?" →"?" →"?" →"?" →"?":bool)
      }
      n362 = for {
        N: 2 -> [_]
        tunnel: w516 -> [w520]
        i -> [w522]
        n363 = Wait (ms)(milliseconds to wait=w520) -> ()  [unwired: 1 out]
        n364 = Equal?(x=0, y=w522) -> (x = y?=→"?" →"?" →"?" →"?" →"?" →"?" →"?" →"?" →"?" →"?":bool)
      }
    }
  }
  n365 = while {
    shift-right: [w563] -> _
    shift-left: "" -> [w565]
    stop <- FALSE stop-if-true
    n366 = event shown="[0] \"Text1\": Value Change" {
      selector: _ -> [_ _ _]
      dyn-events: _ -> [_ _ _]
      timeout: _ -> [_ _ _]
      tunnel: w565 -> [_ _ _]
      tunnel: ["ช่วยด้วย ฉันต้องการความช่วยเหลือ !!!" "ฉันต้องการรับประทานอาหาร" "ฉันมีโรคประจำตัว และรู้สึกอาการกำเริบ !!!"] -> w563
      event "Text1": Value Change {
        n367 = event-data() -> ()  [unwired: 1 in, 6 out]
      }
      event "Text2": Value Change {
        n368 = event-data() -> ()  [unwired: 1 in, 6 out]
      }
      event "Text3": Value Change {
        n369 = event-data() -> ()  [unwired: 1 in, 6 out]
      }
    }
    "String" <- w563
  }
  n370 = call-poly "VISA Configure Serial Port"("VISA resource name"="VISA resource name", "baud rate (9600)"=u32 9600) -> ("VISA resource name out"=w7:refnum<visa-resource-name>, "error out"=w5:errorcluster)  [unwired: 12 in]
  n371 = while {
    shift-right: [w577] -> w6
    shift-left: w7 -> [w578]
    shift-right: [w575] -> w4
    shift-left: w5 -> [w576]
    stop <- FALSE stop-if-true
    n372 = Select(t="a", s="LED", f="b") -> (s? t:f=w572:string)
    n373 = VISA Write(VISA resource name=w578, write buffer=w572, error in (no error)=w576) -> (VISA resource name out=w577:refnum<visa-resource-name>, error out=w575:errorcluster)  [unwired: 1 out]
    n374 = Wait (ms)(milliseconds to wait=u32 5) -> ()  [unwired: 1 out]
  }
  n375 = VISA Close(VISA resource name=w6, error in (no error)=w4) -> ()  [unwired: 1 out]
  n376 = while {
    stop <- FALSE stop-if-true
    n377 = case shown="\"CALL\"" "Tab Control" {
      selector: "Tab Control" -> [w582 w607 w614]
      tunnel: [w581 w606 w612] -> _
      frame "MENU" {
        n378 = local read "Index ที่มากที่สุด"() -> (w587:i32)
        n379 = local read "COMMU"() -> (w588:bool)
        n380 = Add(x=w582, y=3) -> (x+y=w584:u32)
        n381 = local read "Index ที่มากที่สุด"() -> (w596:i32)
        n382 = local read "Index ที่มากที่สุด"() -> (w589:i32)
        n383 = local read "ELEC"() -> (w597:bool)
        n384 = Equal?(x=w587, y=2) -> (x = y?=w590:bool)
        n385 = Increment(x=w582) -> (x+1=w602:enum32{"MENU", "COMMU", "CALL", "ELEC"})
        n386 = local read "CALL"() -> (w593:bool)
        n387 = And(x=w588, y=w590) -> (x .and. y?=w585:bool)
        n388 = Equal?(x=w596, y=0) -> (x = y?=w594:bool)
        n389 = Equal?(x=w589, y=1) -> (x = y?=w591:bool)
        n390 = And(x=w593, y=w591) -> (x .and. y?=w601:bool)
        n391 = And(x=w597, y=w594) -> (x .and. y?=w600:bool)
        n392 = Select(t=w584, s=w585, f=w582) -> (s? t:f=w583:u32)
        n393 = Select(t=w584, s=w601, f=w583) -> (s? t:f=w599:u32)
        n394 = Select(t=w602, s=w600, f=w599) -> (s? t:f=w581:u32)
      }
      frame "COMMU" {
        n395 = local read "Index ที่มากที่สุด"() -> (w610:i32)
        n396 = local read "Back 2"() -> (w605:bool)
        n397 = Decrement(x=w607) -> (x-1=w608:enum32{"MENU", "COMMU", "CALL", "ELEC"})
        n398 = Equal?(x=w610, y=3) -> (x = y?=w604:bool)
        n399 = Not(x=w604) -> (.not. x?=w603:bool)
        n400 = And(x=w605, y=w604) -> (x .and. y?=w611:bool)
        n401 = local write "CALL"(w603) -> ()
        n402 = Select(t=w608, s=w611, f=w607) -> (s? t:f=w606:enum32{"MENU", "COMMU", "CALL", "ELEC"})
      }
      frame "CALL" {
        n403 = local read "Index ที่มากที่สุด"() -> (w620:i32)
        n404 = local read "Back 3"() -> (w613:bool)
        n405 = Subtract(x=w614, y=2) -> (x-y=w615:u32)
        n406 = Equal?(x=w620, y=3) -> (x = y?=w619:bool)
        n407 = Not(x=w619) -> (.not. x?=w618:bool)
        n408 = And(x=w613, y=w619) -> (x .and. y?=w621:bool)
        n409 = local write "CALL"(w618) -> ()
        n410 = Select(t=w615, s=w621, f=w614) -> (s? t:f=w612:u32)
      }
    }
  }
